vi "Plot AxisFocus position.vi"(8 "error in (no error)":errorcluster, 10 "Scale reference":refnum<vi>, 11 "Scale LUT meta":T1) -> (0 "error out":errorcluster)   [LabVIEW 2021, in "RocketPlot.lvlib"]
uses:
  RocketPlot.lvlib
  TypeDefs/Plot scale meta JSON.ctl
  TypeDefs/Plot axis.ctl
  TypeDefs/Plot scale meta state.ctl
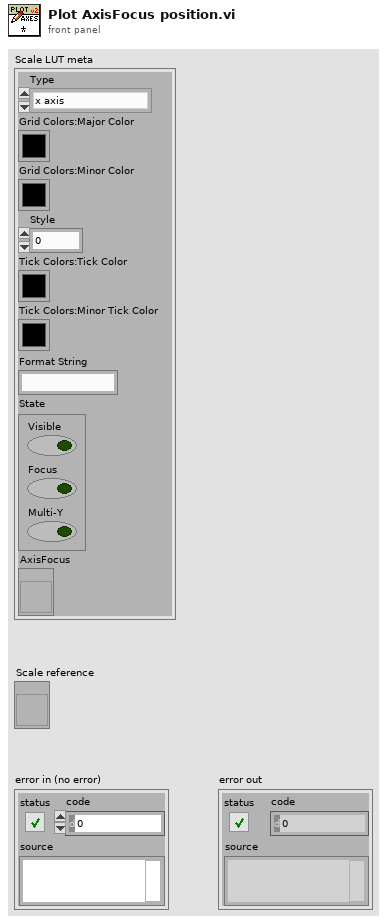
[diagram p1: front panel]
types:
  T1 = typedef "RocketPlot.lvlib/Plot scale meta JSON.ctl" = cluster{"Type":T2, "Grid Colors:Major Color":u32, "Grid Colors:Minor Color":u32, "Style":u8, "Tick Colors:Tick Color":u32, "Tick Colors:Minor Tick Color":u32, "Format String":string, "State":T3, "AxisFocus":refnum<vi>}
  T2 = typedef "RocketPlot.lvlib/Plot axis.ctl" = enum16{"x axis", "left axis", "right axis"}
  T3 = typedef "RocketPlot.lvlib/Plot scale meta state.ctl" = cluster{"Visible":bool, "Focus":bool, "Multi-Y":bool}
  T4 = typedef "LVPositionTypeDef.ctl" = cluster{"Left":i32, "Top":i32}
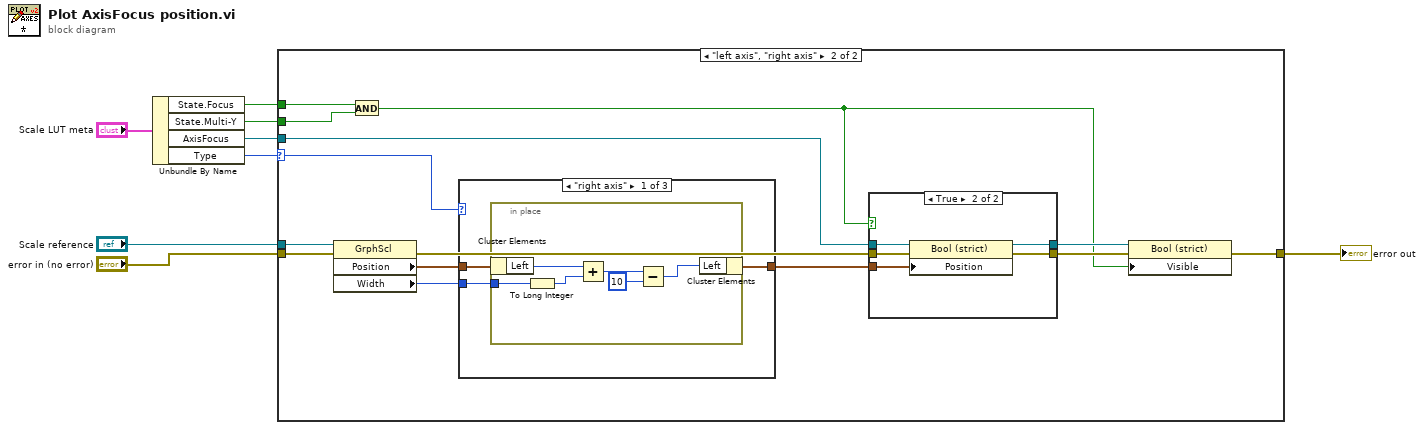
[diagram p0: block diagram]
diagram:
  n1 = Unbundle By Name("Scale LUT meta") -> ("State.Focus"=w8:bool, "State.Multi-Y"=w7:bool, "AxisFocus"=w5:refnum<vi>, "Type"=w1:T2)
  n2 = case shown="\"left axis\", \"right axis\"" w1 {
    selector: w1 -> [_ w14]
    tunnel: w8 -> [_ w23]
    tunnel: w7 -> [_ w22]
    tunnel: w5 -> [_ w13]
    tunnel: "Scale reference" -> [_ w12]
    tunnel: "error in (no error)" -> [w9 w11]
    tunnel: [w9 w10] -> w2
    frame "x axis" {
    }
    frame "left axis", "right axis" {
      n3 = property class="GrphScl"(reference=w12, error in=w11) -> (error out=w17:errorcluster, "Position"=w19:T4, "Width"=w21:u32)  [unwired: 1 out]
      n4 = And(x=w23, y=w22) -> (x .and. y?=w15:bool)
      n5 = case shown="\"right axis\"" w14 {
        tunnel: w19 -> [w26 w33 w34]
        tunnel: [w24 w33 w34] -> w20
        tunnel: w21 -> [w25 _ _]
        frame "right axis" {
          n6 = in-place {
            in-place-border: w25 -> [w28]
            n7 = in-place-cluster #1(w26) -> ("Left"=w32:i32)
            n8 = To Long Integer(number=w28) -> (32bit integer=w27:i32)
            n9 = Add(x=w32, y=w27) -> (x+y=w31:i32)
            n10 = Subtract(x=w31, y=10) -> (x-y=w29:i32)
            n11 = in-place-cluster #1("Left"=w29) -> (w24:T4)
          }
        }
        frame "x axis" {
        }
        frame "left axis" {
        }
      }
      n12 = case shown="True" w15 {
        tunnel: w13 -> [w36 w41]
        tunnel: w20 -> [_ w40]
        tunnel: [w36 w39] -> w16
        tunnel: w17 -> [w35 w38]
        tunnel: [w35 w37] -> w18
        frame False {
        }
        frame True {
          n13 = property class="Bool (strict)"(reference=w41, error in=w38, "Position"=w40) -> (reference out=w39:refnum<vi>, error out=w37:errorcluster)
        }
      }
      n14 = property class="Bool (strict)"(reference=w16, error in=w18, "Visible"=w15) -> (error out=w10:errorcluster)  [unwired: 1 out]
    }
  }
  "error out" <- w2
